vi "changed or first call 1.vi"(1 "timer end":bool, 2 "value":variant) -> (0 "changed or first call?":bool)   [LabVIEW 2019, in "Logik.lvlib"]
uses:
  Logik.lvlib
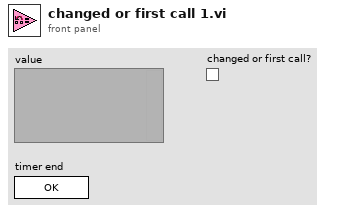
[diagram p1: front panel]
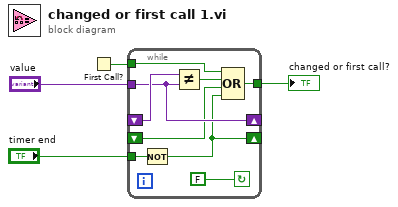
[diagram p0: block diagram]
diagram:
  n1 = First Call?() -> (First Call?: T/F=w4:bool)
  n2 = while {
    tunnel: w4 -> [w8]
    tunnel: [w9] -> w1
    shift-left: _ -> [w13]
    shift-right: [w12] -> _
    tunnel: "value" -> [w12]
    shift-right: [w5] -> _
    shift-left: _ -> [w6]
    tunnel: "timer end" -> [w7]
    stop <- FALSE continue-if-true
    n3 = Not(x=w7) -> (.not. x?=w5:bool)
    n4 = Not Equal?(x=w13, y=w12) -> (x != y?=w11:bool)
    n5 = Compound Arithmetic op=OR(w8, w11, w6, w5) -> (w9:bool)
  }
  "changed or first call?" <- w1
